vi "Main_Console.vi"() -> ()   [LabVIEW 2023]
uses:
  Library/Library_Controls/Order (Z to A).ctl
  Library/Custom_Sort_Library.lvlib
panel:
  in  "Error_In":errorcluster
  out "Error_Out":errorcluster
  out "Table":string[][](table)
  in  "CSV_File_Path":path
  in  "Text_File_Path":path
  in  "Save":bool
  in  "Sort":bool
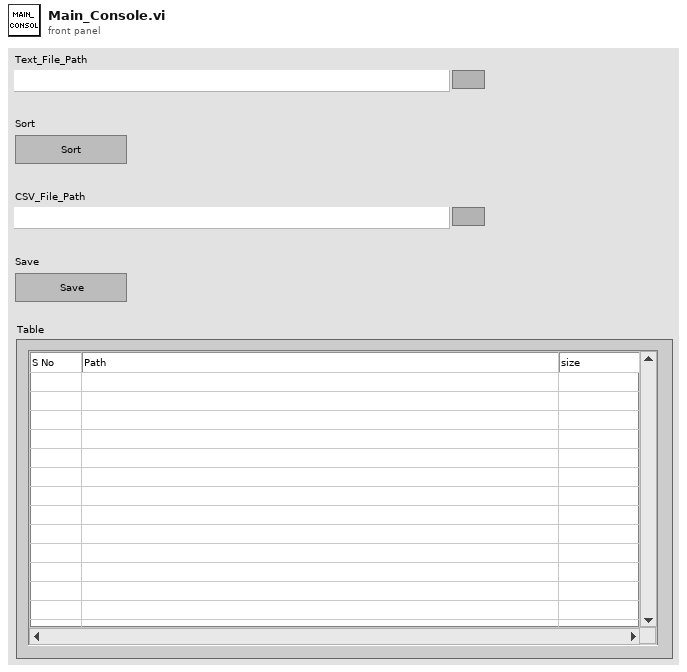
[diagram p1: front panel]
types:
  T1 = typedef "Custom_Sort_Library.lvlib/Order (Z to A).ctl" = enum16{"Z to A", "A to Z"}
  T2 = enum16{"Left Button", "Center Button", "Right Button", "Window Close"}
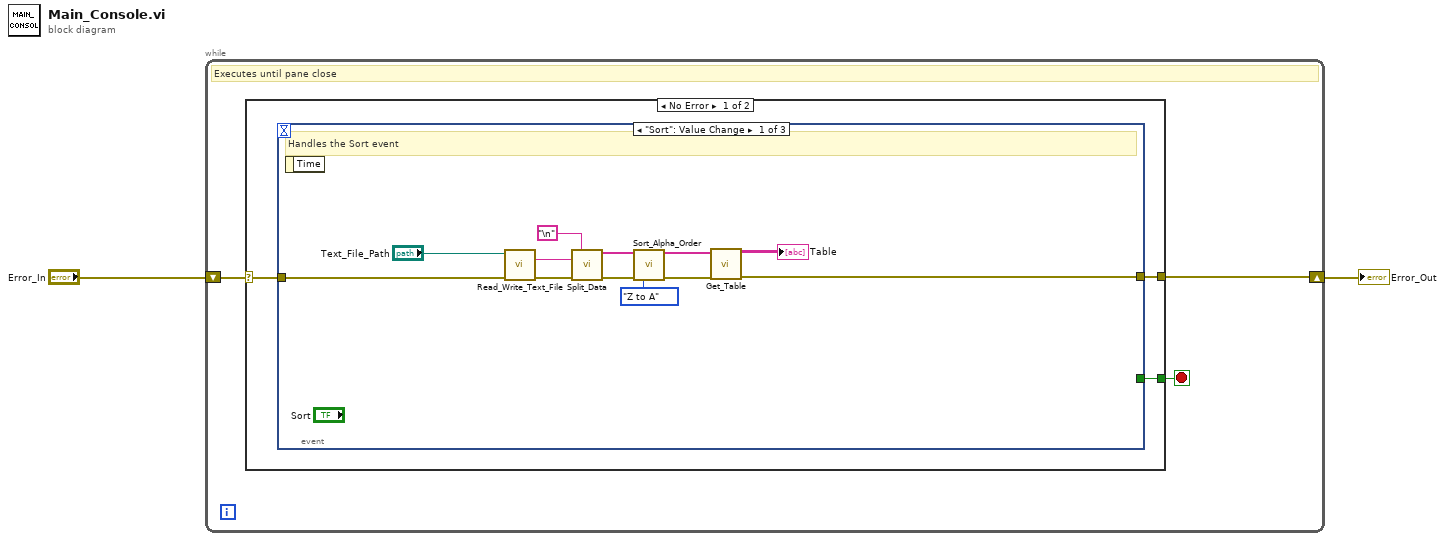
[diagram p0: block diagram]
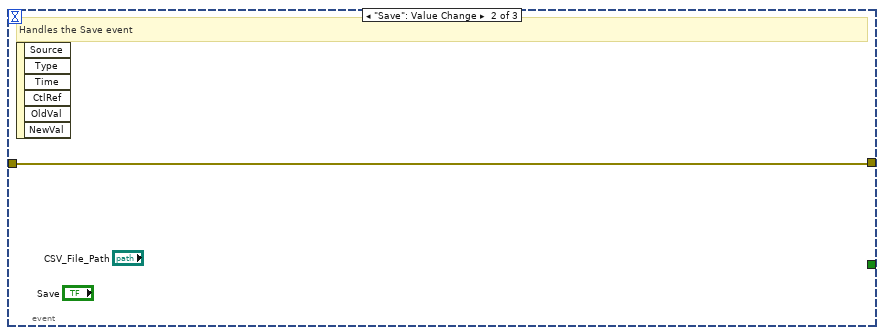
[diagram p2: hidden frame]
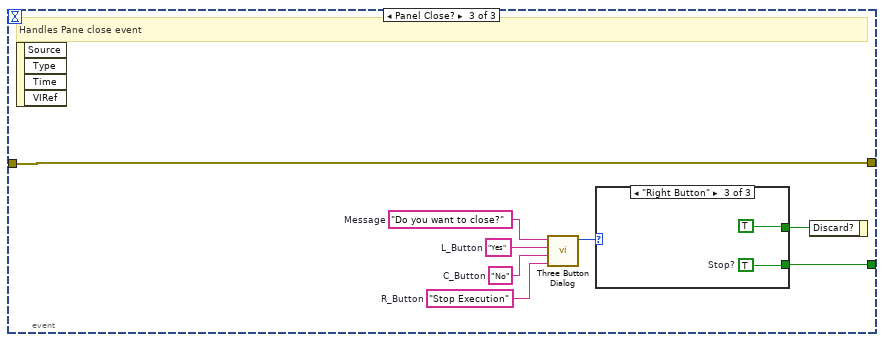
[diagram p3: hidden frame]
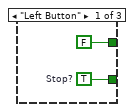
[diagram p4: hidden frame]
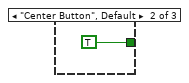
[diagram p5: hidden frame]
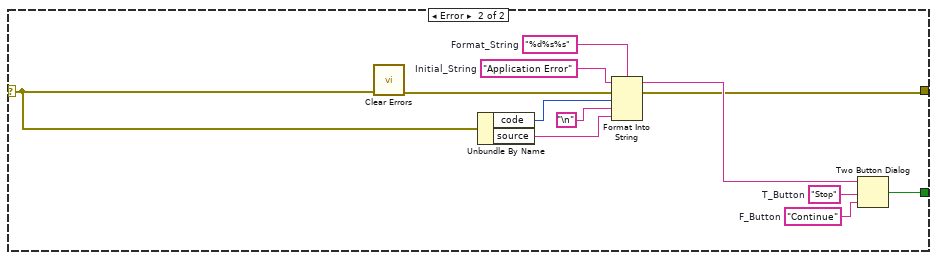
[diagram p6: hidden frame]
diagram:
  n1 = while {
    shift-right: [w4] -> w1
    shift-left: "Error_In" -> [w5]
    stop <- w3 stop-if-true
    # "Executes until pane close"
    n2 = case shown="No Error" w5 {
      selector: w5 -> [w8 w37]
      tunnel: [w7 w36] -> w4
      tunnel: [w6 w35] -> w3
      frame No Error {
        n3 = event shown="[0] \"Sort\": Value Change" {
          selector: _ -> [_ _ _]
          dyn-events: _ -> [_ _ _]
          timeout: _ -> [_ _ _]
          tunnel: w8 -> [w20 w21 w22]
          tunnel: [w9 w21 w22] -> w7
          tunnel: [_ _ w23] -> w6
          event "Sort": Value Change {
            # "Handles the Sort event"
            n4 = event-data() -> ()  [unwired: 1 in, 1 out]
            n5 = call "Read_Write_Text_File.vi"("File_Path_In"="Text_File_Path", "Error_In"=w20) -> ("Data_Out"=w16:string, "Error_Out"=w19:errorcluster)  [unwired: 11 in, 1 out]
            n6 = call "Split_Data.vi"("Delimiter"="\n", "Data_In"=w16, "Error_In"=w19) -> ("Split_Data_Out"=w14:string[], "Error_Out"=w18:errorcluster)  [unwired: 11 in]
            n7 = call "Sort_Alpha_Order.vi"("Split_Data"=w14, "Error_In"=w18, "Order (Z to A)"=Order_(Z_to_A)."Z to A") -> ("Sorted_Array"=w12:string[], "Error_Out"=w10:errorcluster)  [unwired: 11 in]
            n8 = call "Get_Table.vi"("Sorted_Array"=w12, "Error_In"=w10) -> ("Table"=→"Table":string[][], "Error_Out"=w9:errorcluster)  [unwired: 12 in]
          }
          event "Save": Value Change {
            # "Handles the Save event"
            n9 = event-data() -> ()  [unwired: 1 in, 6 out]
          }
          event Panel Close? {
            w26 = "Stop Execution"  # R_Button
            w27 = "No"  # C_Button
            w28 = "Yes"  # L_Button
            w29 = "Do you want to close?"  # Message
            # "Handles Pane close event"
            n10 = event-data() -> ()  [unwired: 1 in, 4 out]
            n11 = call <vilib>:"Three Button Dialog.vi"("Right Button Text (\"Cancel\")"=w26, "Center Button Text (\"No\")"=w27, "Left Button Text (\"Yes\")"=w28, "message"=w29) -> ("Which Button?"=w25:T2)  [unwired: 7 in]
            n12 = case shown="\"Right Button\"" w25 {
              tunnel: [FALSE TRUE TRUE] -> w24
              tunnel: [w30 _ w34] -> w23
              frame "Left Button" {
                w30 = TRUE  # Stop?
              }
              frame "Center Button", Default {
              }
              frame "Right Button" {
                w34 = TRUE  # Stop?
              }
            }
            n13 = event-data("Discard?"=w24) -> ()  [unwired: 1 in, 1 out]
          }
        }
      }
      frame Error {
        w42 = "%d%s%s"  # Format_String
        w43 = "Application Error"  # Initial_String
        w44 = "Stop"  # T_Button
        w45 = "Continue"  # F_Button
        n14 = call <vilib>:"Clear Errors.vi"("error in (no error)"=w37) -> ("error out"=w40:errorcluster)  [unwired: 5 in, 1 out]
        n15 = Unbundle By Name(w37) -> ("code"=w39:i32, "source"=w38:string)
        n16 = Format Into String(format string=w42, initial string=w43, error in=w40, w39, "\n", w38) -> (resulting string=w46:string, error out=w36:errorcluster)
        n17 = Two Button Dialog(message=w46, 1:w45, 2:w44) -> (T button?=w35:bool)
      }
    }
  }
  "Error_Out" <- w1
